vi "Find Safe Cell for King Swap.vi"(9 "Candidate Cells":i32[](array[numeric]), 10 "DT Team #":i32, 11 "1D Board":T1[](array[typedef])) -> (1 "Empty Array?":bool, 2 "Selected Cell":i32, 3 "Safe Cells":i32[](array[numeric]))   [LabVIEW 2014]
uses:
  Typedefs/Board Cell.ctl
  Typedefs/Cell Occupancy.ctl
  Dragon Tamers.lvlib
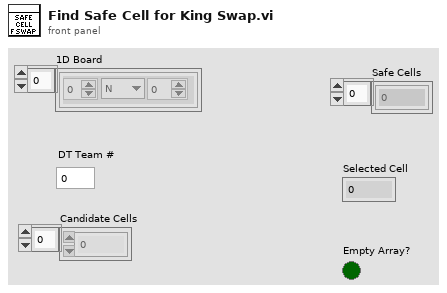
[diagram p1: front panel]
types:
  T1 = typedef "Dragon Tamers.lvlib/Board Cell.ctl" = cluster{"Team":i32, "Occu.":T2, "Count":i32}
  T2 = typedef "Dragon Tamers.lvlib/Cell Occupancy.ctl" = enum16{"N", "C", "K"}
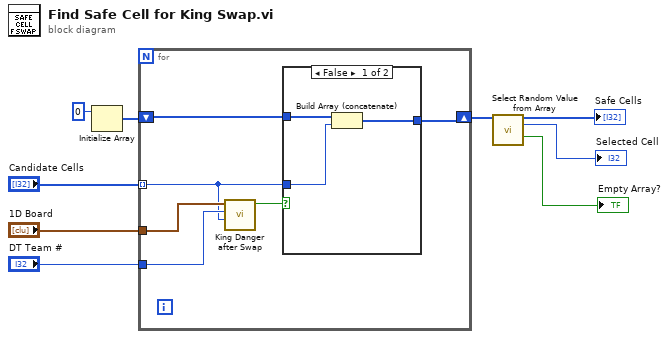
[diagram p0: block diagram]
diagram:
  n1 = Initialize Array(0) -> (w6:i32[])  [unwired: 1 in]
  n2 = for {
    tunnel: "Candidate Cells" -> [w10] mode=indexing
    tunnel: "1D Board" -> [w15]
    tunnel: "DT Team #" -> [w14]
    shift-right: [w11] -> w4
    shift-left: w6 -> [w12]
    n3 = call "King Danger after Swap.vi"("Cell to Swap"=w10, "DT Team #"=w14, "1D Board"=w15) -> ("King in Danger?"=w13:bool)  [unwired: 8 in]
    n4 = case shown="False" w13 {
      tunnel: w12 -> [w18 w19]
      tunnel: [w17 w19] -> w11
      tunnel: w10 -> [w16 _]
      frame False {
        n5 = Build Array (concatenate)(w18, w16) -> (w17:i32[])
      }
      frame True {
      }
    }
  }
  n6 = call "Select Random Value from Array.vi"("Array"=w4) -> ("Array Out"=→"Safe Cells":i32[], "Selected Value"=→"Selected Cell":i32, "Empty Array?"=→"Empty Array?":bool)  [unwired: 11 in, 1 out]
